vi "tb_i12 packingv3.vi"() -> ()   [LabVIEW 2012]
uses:
  ProcessingDLL/Release/ProcessingDLL.dll
panel:
  out "Unpacked LV Version 3":i16[](array[numeric])
  out "Pass3?":bool
  in  "stop":bool
  out "Iteratiosn":i32
  out "Pass2?":bool
  out "Pass?":bool
  out "Unpacked LV Version 2":i16[](array[numeric])
  out "Unpacked LV Version":i16[](array[numeric])
  out "Input 32xI16 Array":i16[](array[numeric])
  # "Input Stimulus"
  # "Output Response"
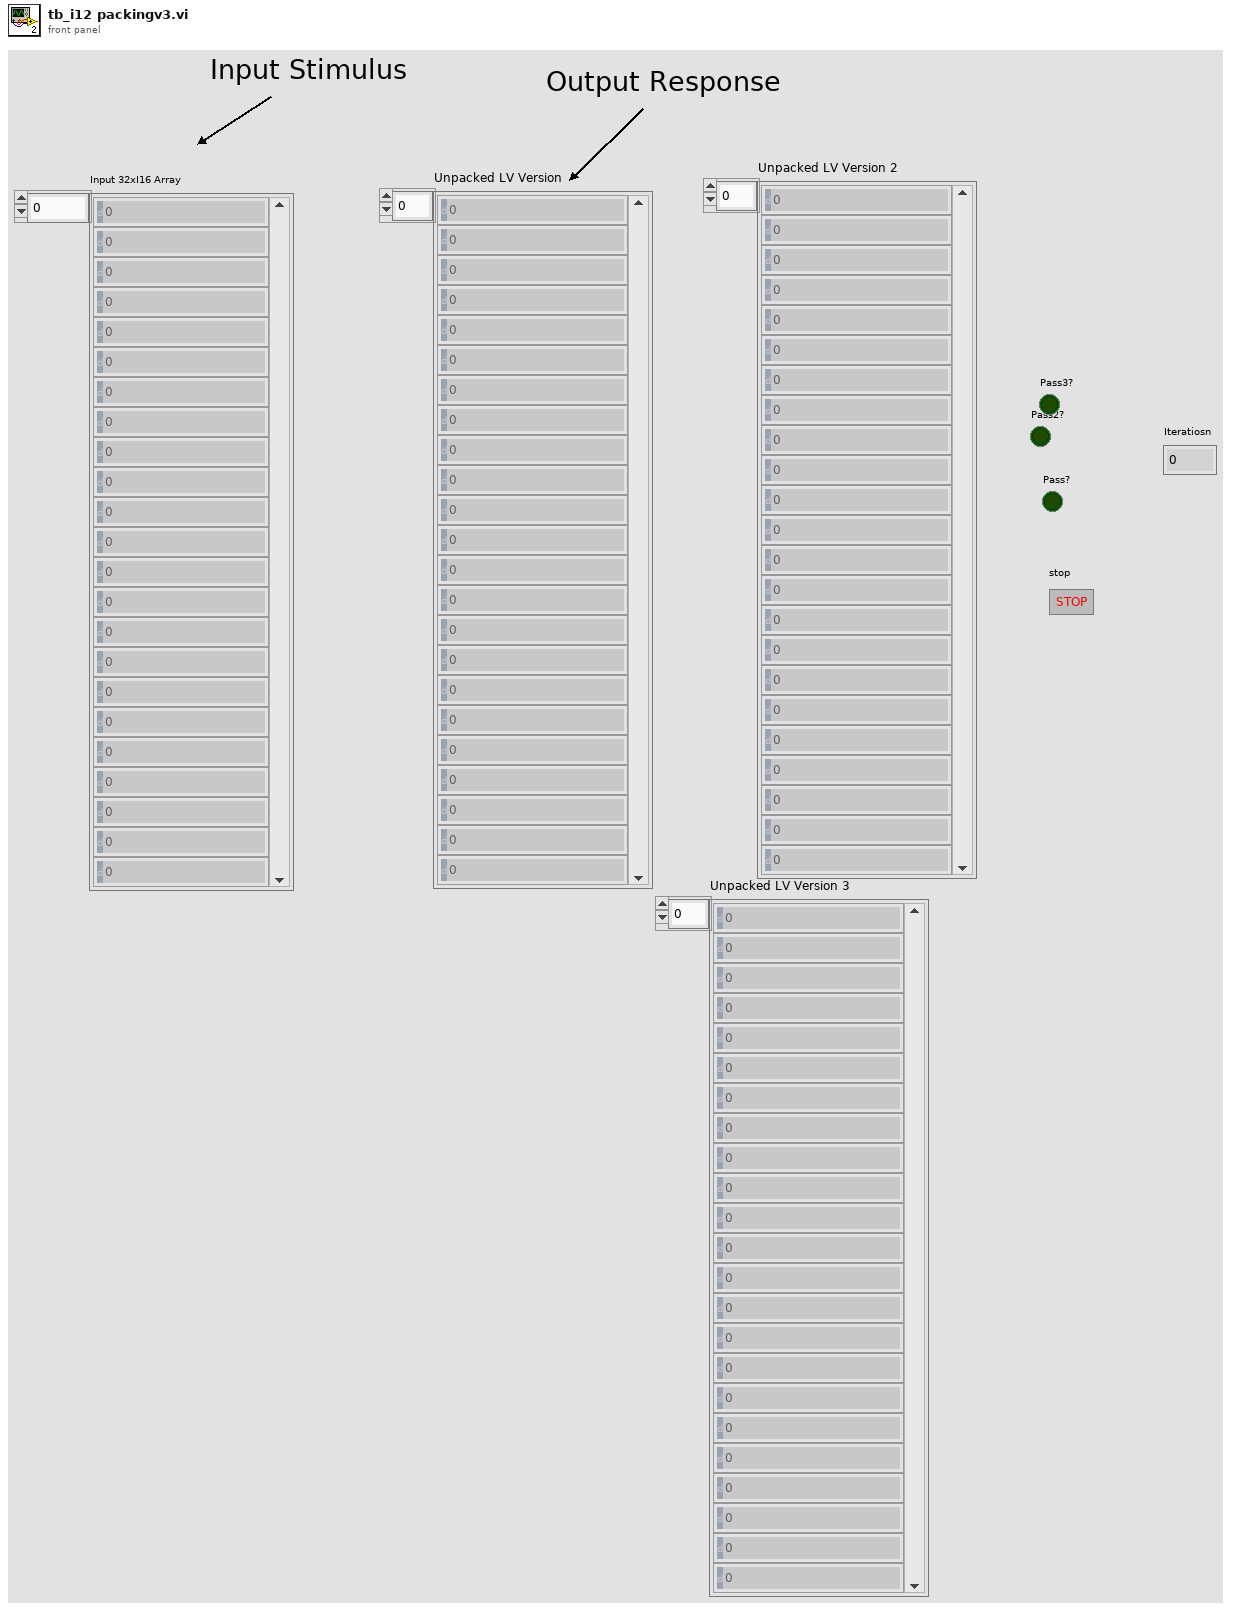
[diagram p1: front panel]
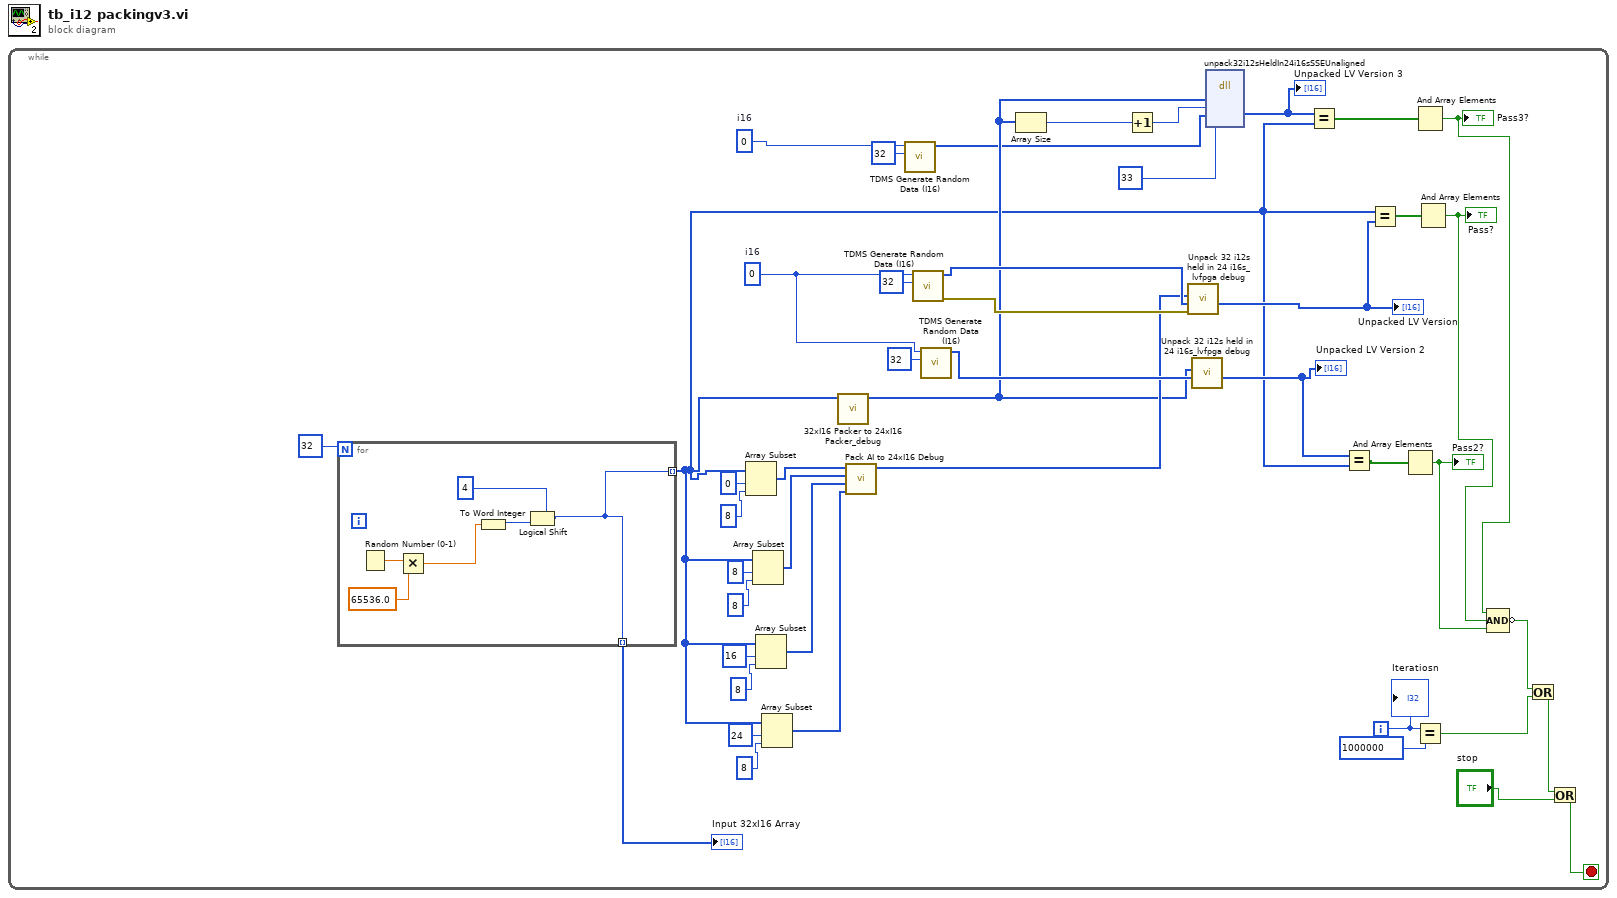
[diagram p0: block diagram]
diagram:
  n1 = while {
    i -> [w17]
    stop <- w12 stop-if-true
    w8 = i16 0  # i16
    w26 = i16 0  # i16
    n2 = for {
      N: 32 -> [_]
      tunnel: [w49] -> w4 mode=indexing
      tunnel: [w49] -> w42 mode=indexing
      n3 = Random Number (0-1)() -> (number: 0 to 1=w48:dbl)
      n4 = Multiply(x=w48, y=65536.0) -> (x*y=w46:dbl)
      n5 = To Word Integer(number=w46) -> (16bit integer=w50:i16)
      n6 = Logical Shift(y=i16 4, x=w50) -> (x << y=w49:i16)
    }
    "Input 32xI16 Array" <- w42
    n7 = Array Subset(array=w4, index=0, length=8 ("index")) -> (w30:i16[])
    n8 = Array Subset(array=w4, index=8, length=8 ("index")) -> (w31:i16[])
    n9 = Array Subset(array=w4, index=16, length=8 ("index")) -> (w32:i16[])
    n10 = Array Subset(array=w4, index=24, length=8 ("index")) -> (w33:i16[])
    n11 = call "32xI16 Packer to 24xI16 Packer_debug.vi"("Input 32xI16 Array"=w4) -> ("Output Data"=w11:i16[])  [unwired: 9 in, 1 out]
    n12 = call "Pack AI to 24xI16 Debug.vi"("Input Set4"=w33, "Input Set3"=w32, "Input Set2"=w31, "Input Set1"=w30) -> ("Output Array"=w23:u16[])  [unwired: 4 in, 3 out]
    n13 = call <vilib>:"TDMS Generate Random Data (I16).vi"("number of samples"=u32 32, "data type"=w8) -> ("data"=w6:i16[])  [unwired: 8 in, 1 out]
    n14 = call <vilib>:"TDMS Generate Random Data (I16).vi"("number of samples"=u32 32, "data type"=w26) -> ("error out"=w43:errorcluster, "data"=w29:i16[])  [unwired: 8 in]
    n15 = call <vilib>:"TDMS Generate Random Data (I16).vi"("number of samples"=u32 32, "data type"=w26) -> ("data"=w27:i16[])  [unwired: 8 in, 1 out]
    n16 = Array Size(array=w11) -> (size(s)=w9:i32)
    n17 = Increment(x=w9) -> (x+1=w10:i32)
    n18 = call "Unpack 32 i12s held in 24 i16s_lvfpga debug.vi"("error in"=w43, "destination i16 array"=w29, "packed i12s"=w23) -> ("destination i16 array out"=w25:i16[])  [unwired: 7 in, 1 out]
    "Unpacked LV Version" <- w25
    n19 = call "Unpack 32 i12s held in 24 i16s_lvfpga debug.vi"("destination i16 array"=w27, "packed i12s"=w11) -> ("destination i16 array out"=w24:i16[])  [unwired: 8 in, 1 out]
    "Unpacked LV Version 2" <- w24
    n20 = dll-call lib="C:/Users/kvemishe/Desktop/LVFPGA Optimized Packer/Test Bench/ProcessingDLL/Release/ProcessingDLL.dll" fn="unpack32i12sHeldIn24i16sSSEUnaligned"("source"=w11, "sourceSize"=w10, "destination"=w6, "destinationSize"=33 ("number of samples")) -> ("destination"=w1:i16[])  [unwired: 7 in, 2 out]
    "Unpacked LV Version 3" <- w1
    n21 = Equal?(x=w1, y=w4) -> (x = y?=w3:bool[])
    n22 = Equal?(x=w24, y=w4) -> (x = y?=w21:bool[])
    n23 = Equal?(x=w4, y=w25) -> (x = y?=w22:bool[])
    n24 = And Array Elements(Boolean array=w21) -> (logical AND=w19:bool)
    "Pass2?" <- w19
    n25 = And Array Elements(Boolean array=w3) -> (logical AND=w2:bool)
    "Pass3?" <- w2
    n26 = Equal?(x=w17, y=1000000) -> (x = y?=w15:bool)
    n27 = And Array Elements(Boolean array=w22) -> (logical AND=w20:bool)
    "Pass?" <- w20
    n28 = Compound Arithmetic op=AND(w2, w20, w19) -> (invert w18:bool)
    n29 = Or(x=w18, y=w15) -> (x .or. y?=w14:bool)
    n30 = Or(x=w14, y="stop") -> (x .or. y?=w12:bool)
    "Iteratiosn" <- w17
  }
